vi "Control Alogrithm.vi"(10 "output cluster":T2, 11 "Voltage Feedback":dbl) -> (3 "Case":u32, 5 "output cluster 2":T1)   [LabVIEW 2019]
panel:
  out "In Range (case 3)":bool
  out "voltage lower(case 1)":bool
  out "voltage higher (case 4)":bool
  out "In Range (case 2)":bool
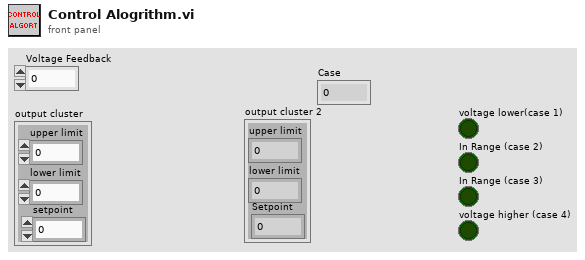
[diagram p1: front panel]
types:
  T1 = cluster{"upper limit":dbl, "lower limit":dbl, "Setpoint":dbl}
  T2 = cluster{"upper limit":dbl, "lower limit":dbl, "setpoint":dbl}
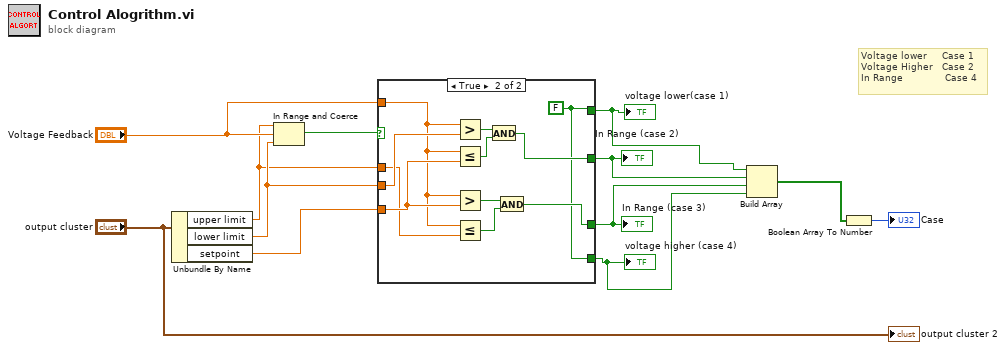
[diagram p0: block diagram]
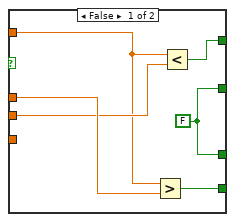
[diagram p2: hidden frame]
diagram:
  # "Voltage lower     Case 1\nVoltage Higher   Case 2 \nIn Range              Case 4"
  n1 = Unbundle By Name("output cluster") -> ("upper limit"=w10:dbl, "lower limit"=w11:dbl, "setpoint"=w6:dbl)
  n2 = In Range and Coerce(upper limit=w10, x="Voltage Feedback", lower limit=w11) -> (In Range?=w9:bool)  [unwired: 1 out]
  n3 = case shown="True" w9 {
    tunnel: w10 -> [w18 w19]
    tunnel: w11 -> [w17 w22]
    tunnel: "Voltage Feedback" -> [w16 w20]
    tunnel: [w13 w24] -> w3
    tunnel: [w13 w25] -> w4
    tunnel: w6 -> [_ w21]
    tunnel: [w15 w23] -> w5
    tunnel: [w14 w23] -> w2
    frame False {
      w13 = FALSE
      n4 = Greater?(x=w16, y=w18) -> (0:w14:bool)
      n5 = Less?(x=w16, y=w17) -> (x < y?=w15:bool)
    }
    frame True {
      w23 = FALSE
      n6 = Greater?(x=w20, y=w22) -> (0:w29:bool)
      n7 = Less Or Equal?(x=w20, y=w21) -> (x <= y?=w28:bool)
      n8 = Greater?(x=w20, y=w21) -> (0:w26:bool)
      n9 = Less Or Equal?(x=w20, y=w19) -> (x <= y?=w27:bool)
      n10 = And(x=w29, y=w28) -> (x .and. y?=w25:bool)
      n11 = And(x=w26, y=w27) -> (x .and. y?=w24:bool)
    }
  }
  "In Range (case 2)" <- w4
  "voltage higher (case 4)" <- w2
  "voltage lower(case 1)" <- w5
  "In Range (case 3)" <- w3
  n12 = Build Array(w5, w4, w3, w2) -> (w1:bool[])
  n13 = Boolean Array To Number(Boolean array=w1) -> (number=→"Case":u32)
  "output cluster 2" <- "output cluster"
